vi "CameraList.vi"(2 "error in":errorcluster, 3 "node":string) -> (0 "error out":errorcluster, 1 "Cameras List":T1)   [LabVIEW 2010]
panel:
  out "Reply":string
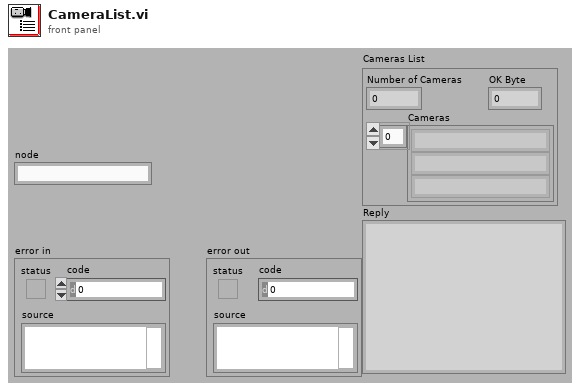
[diagram p1: front panel]
types:
  T1 = cluster{"Number of Cameras":i32, "Cameras":string[], "OK Byte":u8}
  T2 = typedef "_ROSControl.ctl" = cluster{"topic port":u16, "Node":string, "topic":string, "type":string, "node port":u32, "error ":errorcluster, "Direction":T3, "APIs":string[]}
  T3 = typedef "_ROSDirection.ctl" = enum16{"Node", "Publisher", "Subscriber", "Service Client"}
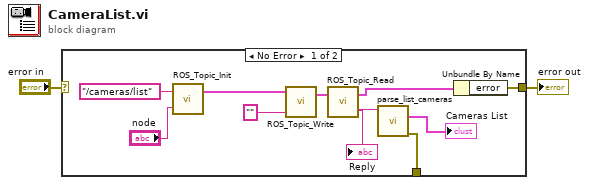
[diagram p0: block diagram]
diagram:
  n1 = case shown="No Error" "error in" {
    selector: "error in" -> [_ w13]
    tunnel: [w12 w13] -> w2
    tunnel: [w3 _] -> _
    frame No Error {
      n2 = call <userlib>:"ROS_Topic_Init.vi"("node"="node", "topic"="/cameras/list") -> ("ROS out"=w10:T2)  [unwired: 1 in]
      n3 = call <userlib>:"ROS_Topic_Write.vi"("Msg in"="", "ROS in"=w10) -> ("ROS out"=w8:T2)  [unwired: 2 in]
      n4 = call <userlib>:"ROS_Topic_Read.vi"("ROS in"=w8) -> ("Reply"=w5:string, "ROS out"=w7:T2)  [unwired: 1 in]
      "Reply" <- w5
      n5 = call <userlib>:"parse_list_cameras.vi"("msg in"=w5) -> ("error out"=w3:errorcluster, "Cameras List"=→"Cameras List":T1)  [unwired: 4 in, 1 out]
      n6 = Unbundle By Name(w7) -> ("error"=w12:errorcluster)
    }
    frame Error {
    }
  }
  "error out" <- w2
